vi "main.vi"() -> ()   [LabVIEW 2023]
panel:
  in  "Conversion\nToggle":bool
  in  "Halt Conversion":bool
  out "Output Temperature":dbl(slide) scale=0.0..300.0
  in  "Input Temperature\nin Celsius":dbl(slide) caption="Input Temperature" scale=0.0..100.0
  # "Fahrenheit"
  # "Celsius"
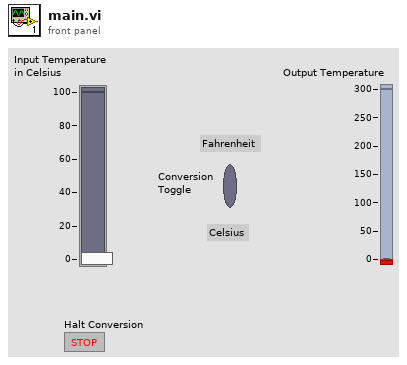
[diagram p1: front panel]
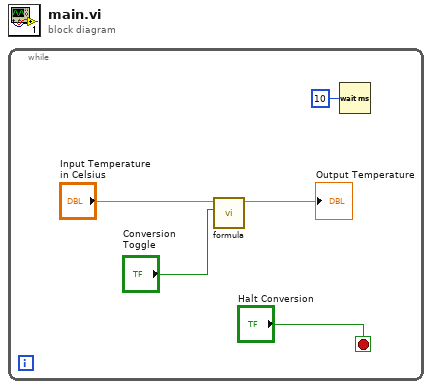
[diagram p0: block diagram]
diagram:
  n1 = while {
    stop <- "Halt Conversion" stop-if-true
    n2 = call "formula.vi"("Conversion\nToggle"="Conversion\nToggle", "Input Temperature\nin Celsius in"="Input Temperature\nin Celsius") -> ("Input Temperature\nin Celsius out"=→"Output Temperature":dbl)  [unwired: 9 in]
    n3 = Wait (ms)(milliseconds to wait=u32 10) -> ()  [unwired: 1 out]
  }
